vi "send_common_trigger.vi"(8 "error in (no error)":errorcluster, 10 "trigger":T1, 11 "GenericToplevelComponent in":refnum<class "GenericToplevelComponent.lvclass">) -> (0 "error out":errorcluster, 3 "GenericToplevelComponent out":refnum<class "GenericToplevelComponent.lvclass">, 4 "# elements in queue":i32)   [LabVIEW 2010, in "GenericToplevelComponent.lvclass"]
uses:
  GenericToplevelComponent.lvclass
  common_trigger_enum.ctl
  trigger_type_enum.ctl
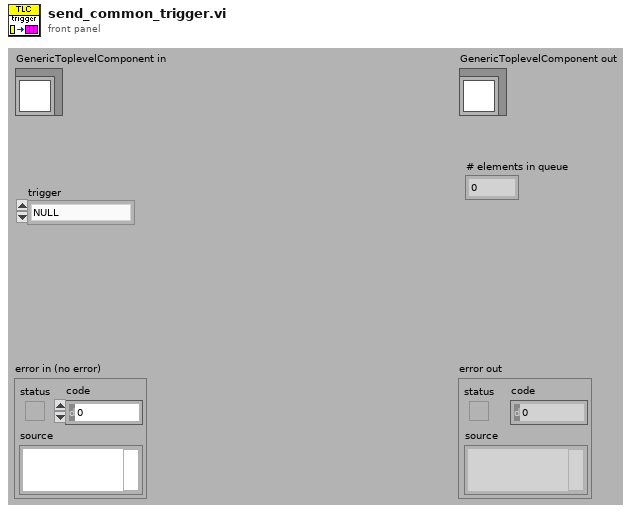
[diagram p1: front panel]
types:
  T1 = typedef "GenericToplevelComponent.lvclass/common_trigger_enum.ctl" = enum16{"NULL", "initialise", "terminate", "fetch command", "fetch data", "attach observer", "register as observer", "detach observer", "acknowledge", "start", "stop", "sweep started", "sweep finished", "experiment started", "experiment stopped"}
  T2 = typedef "trigger_type_enum.ctl" = enum8{"external", "internal", "common"}
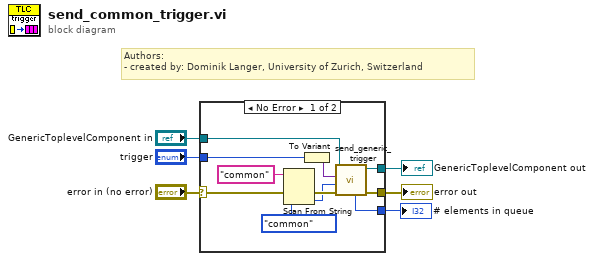
[diagram p0: block diagram]
diagram:
  # "Authors: \n- created by: Dominik Langer, University of Zurich, Switzerland"
  n1 = case shown="No Error" "error in (no error)" {
    selector: "error in (no error)" -> [w11 w19]
    tunnel: [w17 w19] -> w5
    tunnel: [w15 w18] -> w3
    tunnel: "GenericToplevelComponent in" -> [w16 w18]
    tunnel: "trigger" -> [w13 _]
    tunnel: [w12 _] -> w1
    frame No Error {
      n2 = Scan From String(input string="common", error in=w11, default 1=trigger_type_enum."common" ("trigger type")) -> (error out=w10:errorcluster, output 1=w8:T2)  [unwired: 2 in, 2 out]
      n3 = To Variant(anything=w13) -> (Variant=w14:variant)
      n4 = call-dynamic "send_generic_trigger.vi"("error in (no error)"=w10, "trigger type"=w8, "trigger variant"=w14, "GenericToplevelComponent in"=w16) -> ("error out"=w17:errorcluster, "GenericToplevelComponent out"=w15:refnum<class "GenericToplevelComponent.lvclass">, "# elements in queue"=w12:i32)  [unwired: 4 in, 1 out]
    }
    frame Error {
    }
  }
  "error out" <- w5
  "GenericToplevelComponent out" <- w3
  "# elements in queue" <- w1
